vi "UpdateValuesFromDataString.vi"(8 "error In":errorcluster, 10 "New point string":string, 11 "Current String":string) -> (0 "error out":errorcluster, 1 "BG Image":picture, 2 "DisplayString":string, 3 "DataString":string, 4 "WinSize":cluster{"Width":i32, "Height":i32})   [LabVIEW 2023]
doc: "Produces Display String (to be shown) and DataString from current Data string and new data string. \nIf current string starts with lin produces line strings otherwise pos string."
uses:
  StringFormatGlobals.vi
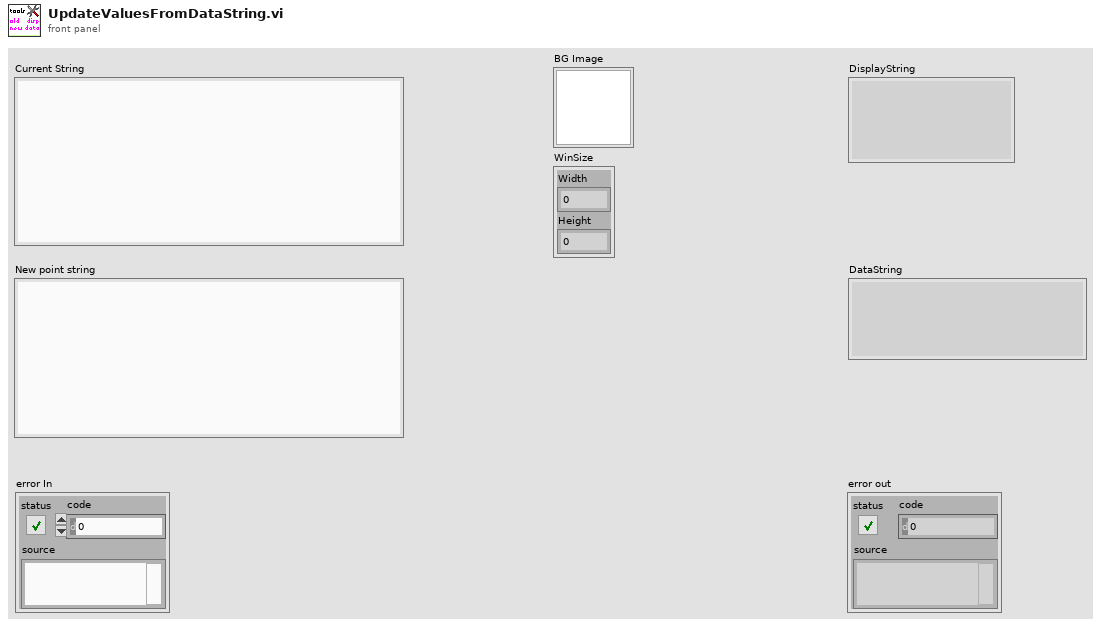
[diagram p1: front panel]
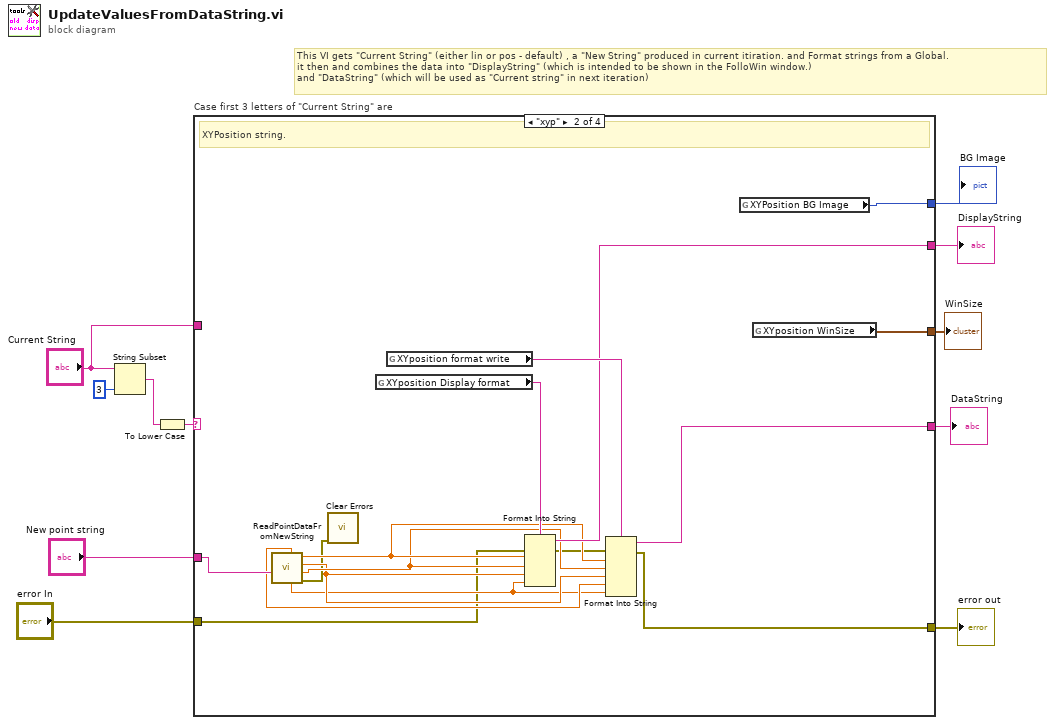
[diagram p0: block diagram]
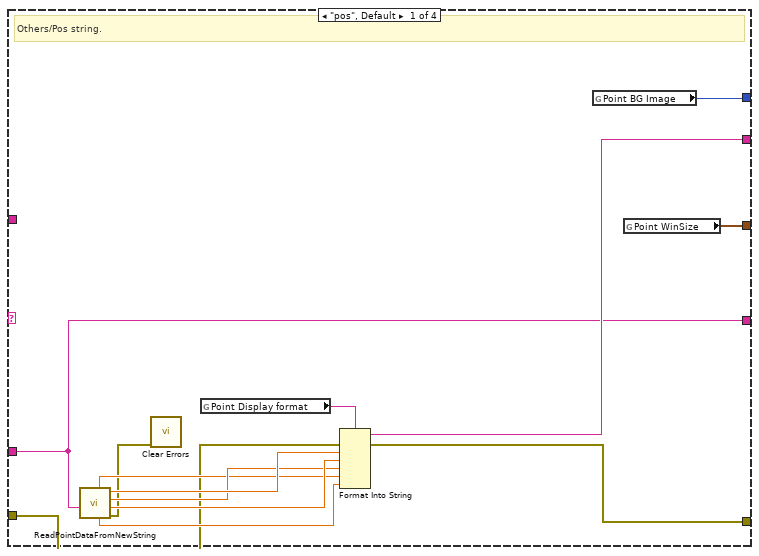
[diagram p2: hidden frame]
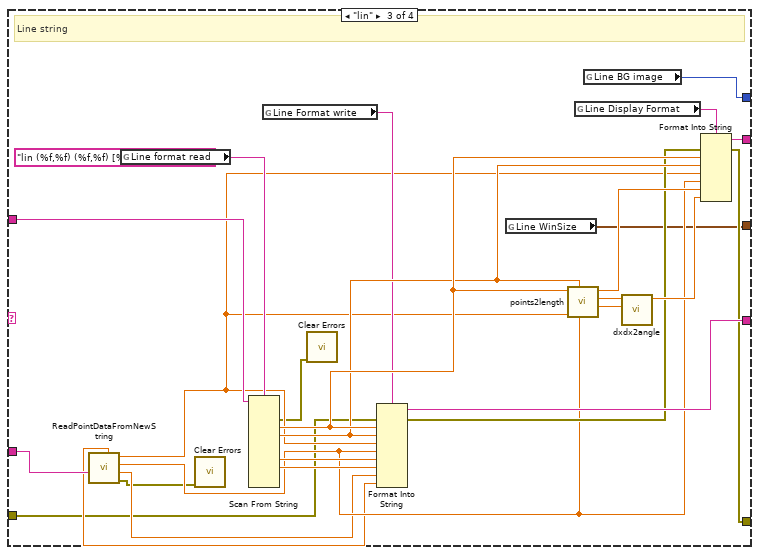
[diagram p3: hidden frame]
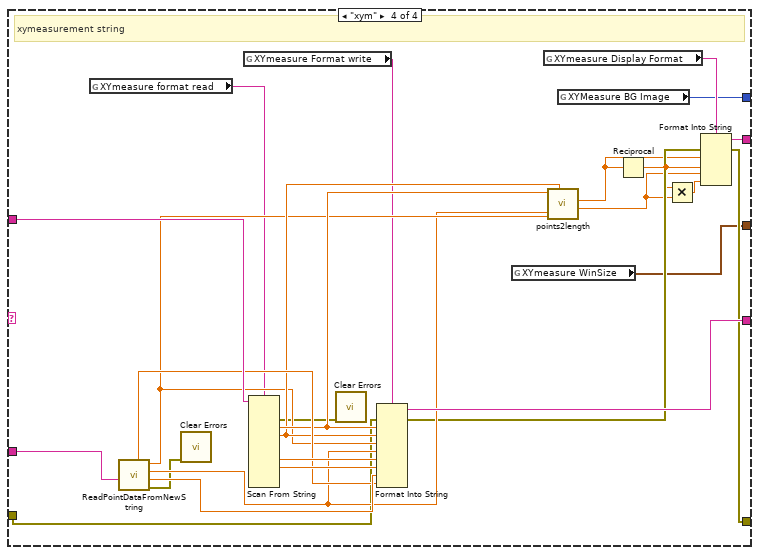
[diagram p4: hidden frame]
diagram:
  # "This VI gets \"Current String\" (either lin or pos - default) , a \"New String\" produced in current itiration. and Format strings from a Global. \nit then and combines the data into \"DisplayString\" (which is intended to be shown in the FolloWin window.) \nand \"DataString\" (which will be used as \"Current string\" in next iteration)"
  n1 = String Subset(string="Current String", length (rest)=3 ("length (rest)")) -> (substring=w10:string)  [unwired: 1 in]
  n2 = To Lower Case(string=w10) -> (all lower case string=w9:string)
  n3 = case "Case first 3 letters of \"Current String\" are" shown="\"xyp\"" w9 {
    tunnel: "Current String" -> [_ _ w66 w92]
    tunnel: "New point string" -> [w17 w36 w50 w91]
    tunnel: [w17 w38 w65 w90] -> w8
    tunnel: [w23 w28 w54 w79] -> w3
    tunnel: "error In" -> [w12 w26 w41 w67]
    tunnel: [w24 w37 w56 w81] -> w4
    tunnel: [w15 w30 w45 w71] -> w2
    tunnel: [w14 w29 w44 w70] -> w1
    frame "pos", Default {
      # "Others/Pos string."
      n4 = call "ReadPointDataFromNewString.vi"("New String"=w17) -> ("error out"=w13:errorcluster, "X index"=w20:dbl, "Y val"=w19:dbl, "X val"=w21:dbl, "Z/F(x)"=w16:dbl, "Y Index"=w18:dbl)  [unwired: 5 in]
      n5 = call <vilib>:"Clear Errors.vi"("error in (no error)"=w13) -> ()  [unwired: 5 in, 2 out]
      n6 = global read "StringFormatGlobals.vi" "Point Display format"() -> (w22:string)
      n7 = Format Into String(format string=w22, error in=w12, w21, w20, w19, w18, w16) -> (resulting string=w24:string, error out=w23:errorcluster)  [unwired: 1 in]
      n8 = global read "StringFormatGlobals.vi" "Point BG Image"() -> (w15:picture)
      n9 = global read "StringFormatGlobals.vi" "Point WinSize"() -> (w14:cluster{"Width":i32, "Height":i32})
    }
    frame "xyp" {
      # "XYPosition string."
      n10 = call "ReadPointDataFromNewString.vi"("New String"=w36) -> ("error out"=w27:errorcluster, "X index"=w34:dbl, "Y val"=w33:dbl, "X val"=w35:dbl, "Z/F(x)"=w31:dbl, "Y Index"=w32:dbl)  [unwired: 5 in]
      n11 = call <vilib>:"Clear Errors.vi"("error in (no error)"=w27) -> ()  [unwired: 5 in, 2 out]
      n12 = global read "StringFormatGlobals.vi" "XYposition Display format"() -> (w40:string)
      n13 = global read "StringFormatGlobals.vi" "XYposition format write"() -> (w39:string)
      n14 = Format Into String(format string=w40, error in=w26, w35, w34, w33, w31) -> (resulting string=w37:string, error out=w25:errorcluster)  [unwired: 1 in]
      n15 = Format Into String(format string=w39, error in=w25, w35, w34, w33, w32, w31) -> (resulting string=w38:string, error out=w28:errorcluster)  [unwired: 1 in]
      n16 = global read "StringFormatGlobals.vi" "XYPosition BG Image"() -> (w30:picture)
      n17 = global read "StringFormatGlobals.vi" "XYposition WinSize"() -> (w29:cluster{"Width":i32, "Height":i32})
    }
    frame "lin" {
      (unwired) "lin (%f,%f) (%f,%f) [%d,%d] [%d,%d]" ("Line format read")
      # "Line string"
      n18 = call "ReadPointDataFromNewString.vi"("New String"=w50) -> ("error out"=w42:errorcluster, "X index"=w47:dbl, "Y val"=w48:dbl, "X val"=w49:dbl, "Y Index"=w46:dbl)  [unwired: 5 in, 1 out]
      n19 = global read "StringFormatGlobals.vi" "Line format read"() -> (w51:string)
      n20 = call <vilib>:"Clear Errors.vi"("error in (no error)"=w42) -> ()  [unwired: 5 in, 2 out]
      n21 = Scan From String(format string=w51, input string=w66) -> (error out=w43:errorcluster, output 1=w60:dbl, output 2=w59:dbl, output 5=w64:dbl, output 6=w63:dbl)  [unwired: 14 in, 2 out]
      n22 = global read "StringFormatGlobals.vi" "Line Format write"() -> (w53:string)
      n23 = call <vilib>:"Clear Errors.vi"("error in (no error)"=w43) -> ()  [unwired: 5 in, 2 out]
      n24 = Format Into String(format string=w53, error in=w41, w60, w59, w49, w48, w64, w63, w47, w46) -> (resulting string=w65:string, error out=w55:errorcluster)  [unwired: 1 in]
      n25 = global read "StringFormatGlobals.vi" "Line WinSize"() -> (w44:cluster{"Width":i32, "Height":i32})
      n26 = call "points2length.vi"("y1"=w48, "y0"=w59, "x1"=w49, "x0"=w60) -> ("dy"=w61:dbl, "dx"=w62:dbl, "Length"=w58:dbl)  [unwired: 4 in, 1 out]
      n27 = global read "StringFormatGlobals.vi" "Line Display Format"() -> (w52:string)
      n28 = global read "StringFormatGlobals.vi" "Line BG image"() -> (w45:picture)
      n29 = call "dxdx2angle.vi"("dy"=w61, "dx"=w62) -> ("Angle Degrees out"=w57:dbl)  [unwired: 8 in, 1 out]
      n30 = Format Into String(format string=w52, error in=w55, w60, w59, w49, w48, w58, w57) -> (resulting string=w56:string, error out=w54:errorcluster)  [unwired: 1 in]
    }
    frame "xym" {
      # "xymeasurement string"
      n31 = global read "StringFormatGlobals.vi" "XYmeasure format read"() -> (w76:string)
      n32 = call "ReadPointDataFromNewString.vi"("New String"=w91) -> ("error out"=w68:errorcluster, "X index"=w87:dbl, "Y val"=w82:dbl, "X val"=w83:dbl, "Y Index"=w86:dbl)  [unwired: 5 in, 1 out]
      n33 = call <vilib>:"Clear Errors.vi"("error in (no error)"=w68) -> ()  [unwired: 5 in, 2 out]
      n34 = global read "StringFormatGlobals.vi" "XYmeasure Format write"() -> (w77:string)
      n35 = Scan From String(format string=w76, input string=w92) -> (error out=w69:errorcluster, output 1=w85:dbl, output 2=w84:dbl, output 5=w89:dbl, output 6=w88:dbl)  [unwired: 14 in, 2 out]
      n36 = call <vilib>:"Clear Errors.vi"("error in (no error)"=w69) -> ()  [unwired: 5 in, 2 out]
      n37 = Format Into String(format string=w77, error in=w67, w85, w84, w83, w82, w89, w88, w87, w86) -> (resulting string=w90:string, error out=w80:errorcluster)  [unwired: 1 in]
      n38 = global read "StringFormatGlobals.vi" "XYmeasure WinSize"() -> (w70:cluster{"Width":i32, "Height":i32})
      n39 = global read "StringFormatGlobals.vi" "XYmeasure Display Format"() -> (w78:string)
      n40 = call "points2length.vi"("y1"=w82, "y0"=w84, "x1"=w83, "x0"=w85) -> ("dy"=w72:dbl, "dx"=w75:dbl)  [unwired: 4 in, 2 out]
      n41 = global read "StringFormatGlobals.vi" "XYMeasure BG Image"() -> (w71:picture)
      n42 = Reciprocal(x=w75) -> (1/x=w73:dbl)
      n43 = Multiply(x=w73, y=w72) -> (x*y=w74:dbl)
      n44 = Format Into String(format string=w78, error in=w80, w75, w73, w72, w74) -> (resulting string=w81:string, error out=w79:errorcluster)  [unwired: 1 in]
    }
  }
  "DataString" <- w8
  "DisplayString" <- w4
  "error out" <- w3
  "BG Image" <- w2
  "WinSize" <- w1
